vi "day 14 task 1.vi"() -> ()   [LabVIEW 2019]
uses:
  48c75094-737f-452e-9833-d8298e23b8a0.vi
panel:
  out "no. units sand come to rest loop":u32
  out "no. units sand come to rest":u32
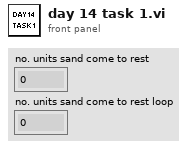
[diagram p1: front panel]
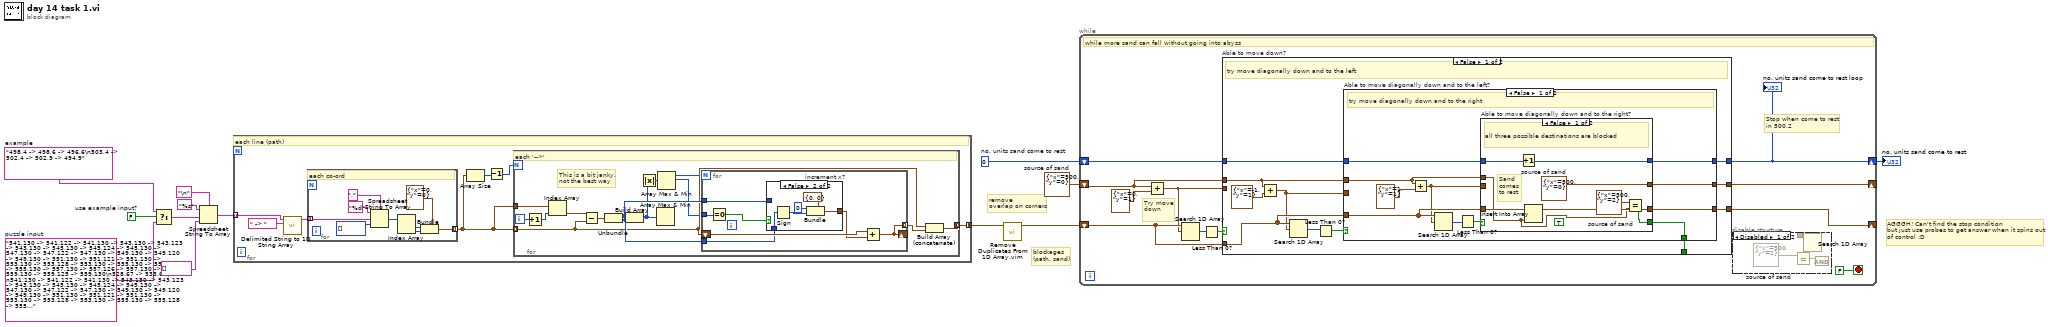
[diagram p0: block diagram]
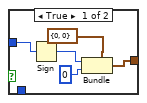
[diagram p6: hidden frame]
diagram:
  w2 = cluster{"x":i32, "y":i32} {"x"=500, "y"=0}  # source of sand
  w3 = u32 0  # no. units sand come to rest
  w8 = FALSE  # use example input?
  w9 = "541,130 -> 541,122 -> 541,130 -> 543,130 -> 543,123 -> 543,130 -> 545,130 -> 545,124 -> 545,130 -> 547,130 -> 547,122 -> 547,130 -> 549,130 -> 549,120 -> 549,130 -> 551,130 -> 551,121 -> 551,130 -> 553,130 -> 553,128 -> 553,130 -> 555,130 -> 555,128 -> 555,130 -> 557,130 -> 557,126 -> 557,130 -> 559,130 -> 559,125 -> 559,130\n528,67 -> 533,67\n541,130 -> 541,122 -> 541,130 -> 543,130 -> 543,123 -> 543,130 -> 545,130 -> 545,124 -> 545,130 -> 547,130 -> 547,122 -> 547,130 -> 549,130 -> 549,120 -> 549,130 -> 551,130 -> 551,121 -> 551,130 -> 553,130 -> 553,128 -> 553,130 -> 555,130 -> 555,128 -> 555,130 -> 557,130 -> 557,126 -> 557,130 -> 559,130 -> 559,125 -> 559,130\n496,23 -> 496,16 -> 496,23 -> 498,23 -> 498,16 -> 498,23 -> 500,23 -> 500,17 -> 500,23 -> 502,23 -> 502,16 -> 502,23\n541,130 -> 541,122 -> 541,130 -> 543,130 -> 543,123 -> 543,130 -> 545,130 -> 545,124 -> 545,130 -> 547,130 -> 547,122 -> 547,130 -> 549,130 -> 549,120 -> 549,130 -> 551,130 -> 551,121 -> 551,130 -> 553,130 -> 553,128 -> 553,130 -> 555,130 -> 555,128 -> 555,130 -> 557,130 -> 557,126 -> 557,130 -> 559,130 -> 559,125 -> 559,130\n514,62 -> 519,62\n509,56 -> 514,56\n497,36 -> 497,30 -> 497,36 -> 499,36 -> 499,27 -> 499,36 -> 501,36 -> 501,33 -> 501,36 -> 503,36 -> 503,27 -> 503,36 -> 505,36 -> 505,28 -> 505,36 -> 507,36 -> 507,35 -> 507,36\n541,130 -> 541,122 -> 541,130 -> 543,130 -> 543,123 -> 543,130 -> 545,130 -> 545,124 -> 545,130 -> 547,130 -> 547,122 -> 547,130 -> 549,130 -> 549,120 -> 549,130 -> 551,130 -> 551,121 -> 551,130 -> 553,130 -> 553,128 -> 553,130 -> 555,130 -> 555,128 -> 555,130 -> 557,130 -> 557,126 -> 557,130 -> 559,130 -> 559,125 -> 559,130\n541,130 -> 541,122 -> 541,130 -> 543,130 -> 543,123 -> 543,130 -> 545,130 -> 545,124 -> 545,130 -> 547,130 -> 547,122 -> 547,130 -> 549,130 -> 549,120 -> 549,130 -> 551,130 -> 551,121 -> 551,130 -> 553,130 -> 553,128 -> 553,130 -> 555,130 -> 555,128 -> 555,130 -> 557,130 -> 557,126 -> 557,130 -> 559,130 -> 559,125 -> 559,130\n574,133 -> 574,137 -> 567,137 -> 567,141 -> 584,141 -> 584,137 -> 576,137 -> 576,133\n524,60 -> 529,60\n574,133 -> 574,137 -> 567,137 -> 567,141 -> 584,141 -> 584,137 -> 576,137 -> 576,133\n541,130 -> 541,122 -> 541,130 -> 543,130 -> 543,123 -> 543,130 -> 545,130 -> 545,124 -> 545,130 -> 547,130 -> 547,122 -> 547,130 -> 549,130 -> 549,120 -> 549,130 -> 551,130 -> 551,121 -> 551,130 -> 553,130 -> 553,128 -> 553,130 -> 555,130 -> 555,128 -> 555,130 -> 557,130 -> 557,126 -> 557,130 -> 559,130 -> 559,125 -> 559,130\n541,130 -> 541,122 -> 541,130 -> 543,130 -> 543,123 -> 543,130 -> 545,130 -> 545,124 -> 545,130 -> 547,130 -> 547,122 -> 547,130 -> 549,130 -> 549,120 -> 549,130 -> 551,130 -> 551,121 -> 551,130 -> 553,130 -> 553,128 -> 553,130 -> 555,130 -> 555,128 -> 555,130 -> 557,130 -> 557,126 -> 557,130 -> 559,130 -> 559,125 -> 559,130\n506,39 -> 506,43 -> 499,43 -> 499,51 -> 514,51 -> 514,43 -> 510,43 -> 510,39\n541,130 -> 541,122 -> 541,130 -> 543,130 -> 543,123 -> 543,130 -> 545,130 -> 545,124 -> 545,130 -> 547,130 -> 547,122 -> 547,130 -> 549,130 -> 549,120 -> 549,130 -> 551,130 -> 551,121 -> 551,130 -> 553,130 -> 553,128 -> 553,130 -> 555,130 -> 555,128 -> 555,130 -> 557,130 -> 557,126 -> 557,130 -> 559,130 -> 559,125 -> 559,130\n541,130 -> 541,122 -> 541,130 -> 543,130 -> 543,123 -> 543,130 -> 545,130 -> 545,124 -> 545,130 -> 547,130 -> 547,122 -> 547,130 -> 549,130 -> 549,120 -> 549,130 -> 551,130 -> 551,121 -> 551,130 -> 553,130 -> 553,128 -> 553,130 -> 555,130 -> 555,128 -> 555,130 -> 557,130 -> 557,126 -> 557,130 -> 559,130 -> 559,125 -> 559,130\n503,60 -> 508,60\n567,115 -> 571,115\n556,151 -> 556,153 -> 548,153 -> 548,157 -> 561,157 -> 561,153 -> 560,153 -> 560,151\n497,36 -> 497,30 -> 497,36 -> 499,36 -> 499,27 -> 499,36 -> 501,36 -> 501,33 -> 501,36 -> 503,36 -> 503,27 -> 503,36 -> 505,36 -> 505,28 -> 505,36 -> 507,36 -> 507,35 -> 507,36\n525,69 -> 530,69\n557,83 -> 557,85 -> 550,85 -> 550,89 -> 569,89 -> 569,85 -> 561,85 -> 561,83\n574,133 -> 574,137 -> 567,137 -> 567,141 -> 584,141 -> 584,137 -> 576,137 -> 576,133\n541,130 -> 541,122 -> 541,130 -> 543,130 -> 543,123 -> 543,130 -> 545,130 -> 545,124 -> 545,130 -> 547,130 -> 547,122 -> 547,130 -> 549,130 -> 549,120 -> 549,130 -> 551,130 -> 551,121 -> 551,130 -> 553,130 -> 553,128 -> 553,130 -> 555,130 -> 555,128 -> 555,130 -> 557,130 -> 557,126 -> 557,130 -> 559,130 -> 559,125 -> 559,130\n496,23 -> 496,16 -> 496,23 -> 498,23 -> 498,16 -> 498,23 -> 500,23 -> 500,17 -> 500,23 -> 502,23 -> 502,16 -> 502,23\n564,108 -> 564,107 -> 564,108 -> 566,108 -> 566,101 -> 566,108 -> 568,108 -> 568,100 -> 568,108\n496,23 -> 496,16 -> 496,23 -> 498,23 -> 498,16 -> 498,23 -> 500,23 -> 500,17 -> 500,23 -> 502,23 -> 502,16 -> 502,23\n556,151 -> 556,153 -> 548,153 -> 548,157 -> 561,157 -> 561,153 -> 560,153 -> 560,151\n541,130 -> 541,122 -> 541,130 -> 543,130 -> 543,123 -> 543,130 -> 545,130 -> 545,124 -> 545,130 -> 547,130 -> 547,122 -> 547,130 -> 549,130 -> 549,120 -> 549,130 -> 551,130 -> 551,121 -> 551,130 -> 553,130 -> 553,128 -> 553,130 -> 555,130 -> 555,128 -> 555,130 -> 557,130 -> 557,126 -> 557,130 -> 559,130 -> 559,125 -> 559,130\n497,36 -> 497,30 -> 497,36 -> 499,36 -> 499,27 -> 499,36 -> 501,36 -> 501,33 -> 501,36 -> 503,36 -> 503,27 -> 503,36 -> 505,36 -> 505,28 -> 505,36 -> 507,36 -> 507,35 -> 507,36\n556,151 -> 556,153 -> 548,153 -> 548,157 -> 561,157 -> 561,153 -> 560,153 -> 560,151\n561,115 -> 565,115\n564,144 -> 568,144\n497,36 -> 497,30 -> 497,36 -> 499,36 -> 499,27 -> 499,36 -> 501,36 -> 501,33 -> 501,36 -> 503,36 -> 503,27 -> 503,36 -> 505,36 -> 505,28 -> 505,36 -> 507,36 -> 507,35 -> 507,36\n541,130 -> 541,122 -> 541,130 -> 543,130 -> 543,123 -> 543,130 -> 545,130 -> 545,124 -> 545,130 -> 547,130 -> 547,122 -> 547,130 -> 549,130 -> 549,120 -> 549,130 -> 551,130 -> 551,121 -> 551,130 -> 553,130 -> 553,128 -> 553,130 -> 555,130 -> 555,128 -> 555,130 -> 557,130 -> 557,126 -> 557,130 -> 559,130 -> 559,125 -> 559,130\n497,36 -> 497,30 -> 497,36 -> 499,36 -> 499,27 -> 499,36 -> 501,36 -> 501,33 -> 501,36 -> 503,36 -> 503,27 -> 503,36 -> 505,36 -> 505,28 -> 505,36 -> 507,36 -> 507,35 -> 507,36\n556,151 -> 556,153 -> 548,153 -> 548,157 -> 561,157 -> 561,153 -> 560,153 -> 560,151\n557,83 -> 557,85 -> 550,85 -> 550,89 -> 569,89 -> 569,85 -> 561,85 -> 561,83\n496,23 -> 496,16 -> 496,23 -> 498,23 -> 498,16 -> 498,23 -> 500,23 -> 500,17 -> 500,23 -> 502,23 -> 502,16 -> 502,23\n567,146 -> 571,146\n531,65 -> 536,65\n528,62 -> 533,62\n541,130 -> 541,122 -> 541,130 -> 543,130 -> 543,123 -> 543,130 -> 545,130 -> 545,124 -> 545,130 -> 547,130 -> 547,122 -> 547,130 -> 549,130 -> 549,120 -> 549,130 -> 551,130 -> 551,121 -> 551,130 -> 553,130 -> 553,128 -> 553,130 -> 555,130 -> 555,128 -> 555,130 -> 557,130 -> 557,126 -> 557,130 -> 559,130 -> 559,125 -> 559,130\n541,130 -> 541,122 -> 541,130 -> 543,130 -> 543,123 -> 543,130 -> 545,130 -> 545,124 -> 545,130 -> 547,130 -> 547,122 -> 547,130 -> 549,130 -> 549,120 -> 549,130 -> 551,130 -> 551,121 -> 551,130 -> 553,130 -> 553,128 -> 553,130 -> 555,130 -> 555,128 -> 555,130 -> 557,130 -> 557,126 -> 557,130 -> 559,130 -> 559,125 -> 559,130\n574,133 -> 574,137 -> 567,137 -> 567,141 -> 584,141 -> 584,137 -> 576,137 -> 576,133\n568,95 -> 571,95 -> 571,94\n497,36 -> 497,30 -> 497,36 -> 499,36 -> 499,27 -> 499,36 -> 501,36 -> 501,33 -> 501,36 -> 503,36 -> 503,27 -> 503,36 -> 505,36 -> 505,28 -> 505,36 -> 507,36 -> 507,35 -> 507,36\n497,36 -> 497,30 -> 497,36 -> 499,36 -> 499,27 -> 499,36 -> 501,36 -> 501,33 -> 501,36 -> 503,36 -> 503,27 -> 503,36 -> 505,36 -> 505,28 -> 505,36 -> 507,36 -> 507,35 -> 507,36\n497,36 -> 497,30 -> 497,36 -> 499,36 -> 499,27 -> 499,36 -> 501,36 -> 501,33 -> 501,36 -> 503,36 -> 503,27 -> 503,36 -> 505,36 -> 505,28 -> 505,36 -> 507,36 -> 507,35 -> 507,36\n541,130 -> 541,122 -> 541,130 -> 543,130 -> 543,123 -> 543,130 -> 545,130 -> 545,124 -> 545,130 -> 547,130 -> 547,122 -> 547,130 -> 549,130 -> 549,120 -> 549,130 -> 551,130 -> 551,121 -> 551,130 -> 553,130 -> 553,128 -> 553,130 -> 555,130 -> 555,128 -> 555,130 -> 557,130 -> 557,126 -> 557,130 -> 559,130 -> 559,125 -> 559,130\n557,83 -> 557,85 -> 550,85 -> 550,89 -> 569,89 -> 569,85 -> 561,85 -> 561,83\n543,72 -> 543,73 -> 554,73 -> 554,72\n506,39 -> 506,43 -> 499,43 -> 499,51 -> 514,51 -> 514,43 -> 510,43 -> 510,39\n555,115 -> 559,115\n496,23 -> 496,16 -> 496,23 -> 498,23 -> 498,16 -> 498,23 -> 500,23 -> 500,17 -> 500,23 -> 502,23 -> 502,16 -> 502,23\n506,39 -> 506,43 -> 499,43 -> 499,51 -> 514,51 -> 514,43 -> 510,43 -> 510,39\n536,75 -> 536,76 -> 547,76 -> 547,75\n521,62 -> 526,62\n564,108 -> 564,107 -> 564,108 -> 566,108 -> 566,101 -> 566,108 -> 568,108 -> 568,100 -> 568,108\n574,133 -> 574,137 -> 567,137 -> 567,141 -> 584,141 -> 584,137 -> 576,137 -> 576,133\n516,56 -> 521,56\n564,108 -> 564,107 -> 564,108 -> 566,108 -> 566,101 -> 566,108 -> 568,108 -> 568,100 -> 568,108\n543,72 -> 543,73 -> 554,73 -> 554,72\n574,133 -> 574,137 -> 567,137 -> 567,141 -> 584,141 -> 584,137 -> 576,137 -> 576,133\n564,113 -> 568,113\n506,39 -> 506,43 -> 499,43 -> 499,51 -> 514,51 -> 514,43 -> 510,43 -> 510,39\n541,130 -> 541,122 -> 541,130 -> 543,130 -> 543,123 -> 543,130 -> 545,130 -> 545,124 -> 545,130 -> 547,130 -> 547,122 -> 547,130 -> 549,130 -> 549,120 -> 549,130 -> 551,130 -> 551,121 -> 551,130 -> 553,130 -> 553,128 -> 553,130 -> 555,130 -> 555,128 -> 555,130 -> 557,130 -> 557,126 -> 557,130 -> 559,130 -> 559,125 -> 559,130\n496,23 -> 496,16 -> 496,23 -> 498,23 -> 498,16 -> 498,23 -> 500,23 -> 500,17 -> 500,23 -> 502,23 -> 502,16 -> 502,23\n557,83 -> 557,85 -> 550,85 -> 550,89 -> 569,89 -> 569,85 -> 561,85 -> 561,83\n558,113 -> 562,113\n497,36 -> 497,30 -> 497,36 -> 499,36 -> 499,27 -> 499,36 -> 501,36 -> 501,33 -> 501,36 -> 503,36 -> 503,27 -> 503,36 -> 505,36 -> 505,28 -> 505,36 -> 507,36 -> 507,35 -> 507,36\n506,39 -> 506,43 -> 499,43 -> 499,51 -> 514,51 -> 514,43 -> 510,43 -> 510,39\n497,36 -> 497,30 -> 497,36 -> 499,36 -> 499,27 -> 499,36 -> 501,36 -> 501,33 -> 501,36 -> 503,36 -> 503,27 -> 503,36 -> 505,36 -> 505,28 -> 505,36 -> 507,36 -> 507,35 -> 507,36\n568,95 -> 571,95 -> 571,94\n497,36 -> 497,30 -> 497,36 -> 499,36 -> 499,27 -> 499,36 -> 501,36 -> 501,33 -> 501,36 -> 503,36 -> 503,27 -> 503,36 -> 505,36 -> 505,28 -> 505,36 -> 507,36 -> 507,35 -> 507,36\n510,60 -> 515,60\n497,36 -> 497,30 -> 497,36 -> 499,36 -> 499,27 -> 499,36 -> 501,36 -> 501,33 -> 501,36 -> 503,36 -> 503,27 -> 503,36 -> 505,36 -> 505,28 -> 505,36 -> 507,36 -> 507,35 -> 507,36\n557,83 -> 557,85 -> 550,85 -> 550,89 -> 569,89 -> 569,85 -> 561,85 -> 561,83\n570,117 -> 574,117\n497,36 -> 497,30 -> 497,36 -> 499,36 -> 499,27 -> 499,36 -> 501,36 -> 501,33 -> 501,36 -> 503,36 -> 503,27 -> 503,36 -> 505,36 -> 505,28 -> 505,36 -> 507,36 -> 507,35 -> 507,36\n507,62 -> 512,62\n541,130 -> 541,122 -> 541,130 -> 543,130 -> 543,123 -> 543,130 -> 545,130 -> 545,124 -> 545,130 -> 547,130 -> 547,122 -> 547,130 -> 549,130 -> 549,120 -> 549,130 -> 551,130 -> 551,121 -> 551,130 -> 553,130 -> 553,128 -> 553,130 -> 555,130 -> 555,128 -> 555,130 -> 557,130 -> 557,126 -> 557,130 -> 559,130 -> 559,125 -> 559,130\n556,151 -> 556,153 -> 548,153 -> 548,157 -> 561,157 -> 561,153 -> 560,153 -> 560,151\n564,108 -> 564,107 -> 564,108 -> 566,108 -> 566,101 -> 566,108 -> 568,108 -> 568,100 -> 568,108\n541,130 -> 541,122 -> 541,130 -> 543,130 -> 543,123 -> 543,130 -> 545,130 -> 545,124 -> 545,130 -> 547,130 -> 547,122 -> 547,130 -> 549,130 -> 549,120 -> 549,130 -> 551,130 -> 551,121 -> 551,130 -> 553,130 -> 553,128 -> 553,130 -> 555,130 -> 555,128 -> 555,130 -> 557,130 -> 557,126 -> 557,130 -> 559,130 -> 559,125 -> 559,130\n506,39 -> 506,43 -> 499,43 -> 499,51 -> 514,51 -> 514,43 -> 510,43 -> 510,39\n564,108 -> 564,107 -> 564,108 -> 566,108 -> 566,101 -> 566,108 -> 568,108 -> 568,100 -> 568,108\n497,36 -> 497,30 -> 497,36 -> 499,36 -> 499,27 -> 499,36 -> 501,36 -> 501,33 -> 501,36 -> 503,36 -> 503,27 -> 503,36 -> 505,36 -> 505,28 -> 505,36 -> 507,36 -> 507,35 -> 507,36\n561,111 -> 565,111\n541,130 -> 541,122 -> 541,130 -> 543,130 -> 543,123 -> 543,130 -> 545,130 -> 545,124 -> 545,130 -> 547,130 -> 547,122 -> 547,130 -> 549,130 -> 549,120 -> 549,130 -> 551,130 -> 551,121 -> 551,130 -> 553,130 -> 553,128 -> 553,130 -> 555,130 -> 555,128 -> 555,130 -> 557,130 -> 557,126 -> 557,130 -> 559,130 -> 559,125 -> 559,130\n541,130 -> 541,122 -> 541,130 -> 543,130 -> 543,123 -> 543,130 -> 545,130 -> 545,124 -> 545,130 -> 547,130 -> 547,122 -> 547,130 -> 549,130 -> 549,120 -> 549,130 -> 551,130 -> 551,121 -> 551,130 -> 553,130 -> 553,128 -> 553,130 -> 555,130 -> 555,128 -> 555,130 -> 557,130 -> 557,126 -> 557,130 -> 559,130 -> 559,125 -> 559,130\n541,130 -> 541,122 -> 541,130 -> 543,130 -> 543,123 -> 543,130 -> 545,130 -> 545,124 -> 545,130 -> 547,130 -> 547,122 -> 547,130 -> 549,130 -> 549,120 -> 549,130 -> 551,130 -> 551,121 -> 551,130 -> 553,130 -> 553,128 -> 553,130 -> 555,130 -> 555,128 -> 555,130 -> 557,130 -> 557,126 -> 557,130 -> 559,130 -> 559,125 -> 559,130\n496,23 -> 496,16 -> 496,23 -> 498,23 -> 498,16 -> 498,23 -> 500,23 -> 500,17 -> 500,23 -> 502,23 -> 502,16 -> 502,23\n558,148 -> 562,148\n513,58 -> 518,58\n564,108 -> 564,107 -> 564,108 -> 566,108 -> 566,101 -> 566,108 -> 568,108 -> 568,100 -> 568,108\n558,117 -> 562,117\n557,83 -> 557,85 -> 550,85 -> 550,89 -> 569,89 -> 569,85 -> 561,85 -> 561,83\n546,79 -> 546,80 -> 558,80\n541,130 -> 541,122 -> 541,130 -> 543,130 -> 543,123 -> 543,130 -> 545,130 -> 545,124 -> 545,130 -> 547,130 -> 547,122 -> 547,130 -> 549,130 -> 549,120 -> 549,130 -> 551,130 -> 551,121 -> 551,130 -> 553,130 -> 553,128 -> 553,130 -> 555,130 -> 555,128 -> 555,130 -> 557,130 -> 557,126 -> 557,130 -> 559,130 -> 559,125 -> 559,130\n541,130 -> 541,122 -> 541,130 -> 543,130 -> 543,123 -> 543,130 -> 545,130 -> 545,124 -> 545,130 -> 547,130 -> 547,122 -> 547,130 -> 549,130 -> 549,120 -> 549,130 -> 551,130 -> 551,121 -> 551,130 -> 553,130 -> 553,128 -> 553,130 -> 555,130 -> 555,128 -> 555,130 -> 557,130 -> 557,126 -> 557,130 -> 559,130 -> 559,125 -> 559,130\n536,75 -> 536,76 -> 547,76 -> 547,75\n500,62 -> 505,62\n506,39 -> 506,43 -> 499,43 -> 499,51 -> 514,51 -> 514,43 -> 510,43 -> 510,39\n556,151 -> 556,153 -> 548,153 -> 548,157 -> 561,157 -> 561,153 -> 560,153 -> 560,151\n520,58 -> 525,58\n535,67 -> 540,67\n574,133 -> 574,137 -> 567,137 -> 567,141 -> 584,141 -> 584,137 -> 576,137 -> 576,133\n497,36 -> 497,30 -> 497,36 -> 499,36 -> 499,27 -> 499,36 -> 501,36 -> 501,33 -> 501,36 -> 503,36 -> 503,27 -> 503,36 -> 505,36 -> 505,28 -> 505,36 -> 507,36 -> 507,35 -> 507,36\n541,130 -> 541,122 -> 541,130 -> 543,130 -> 543,123 -> 543,130 -> 545,130 -> 545,124 -> 545,130 -> 547,130 -> 547,122 -> 547,130 -> 549,130 -> 549,120 -> 549,130 -> 551,130 -> 551,121 -> 551,130 -> 553,130 -> 553,128 -> 553,130 -> 555,130 -> 555,128 -> 555,130 -> 557,130 -> 557,126 -> 557,130 -> 559,130 -> 559,125 -> 559,130\n546,79 -> 546,80 -> 558,80\n564,108 -> 564,107 -> 564,108 -> 566,108 -> 566,101 -> 566,108 -> 568,108 -> 568,100 -> 568,108\n543,72 -> 543,73 -> 554,73 -> 554,72\n564,117 -> 568,117\n497,36 -> 497,30 -> 497,36 -> 499,36 -> 499,27 -> 499,36 -> 501,36 -> 501,33 -> 501,36 -> 503,36 -> 503,27 -> 503,36 -> 505,36 -> 505,28 -> 505,36 -> 507,36 -> 507,35 -> 507,36\n497,36 -> 497,30 -> 497,36 -> 499,36 -> 499,27 -> 499,36 -> 501,36 -> 501,33 -> 501,36 -> 503,36 -> 503,27 -> 503,36 -> 505,36 -> 505,28 -> 505,36 -> 507,36 -> 507,35 -> 507,36\n536,75 -> 536,76 -> 547,76 -> 547,75\n557,83 -> 557,85 -> 550,85 -> 550,89 -> 569,89 -> 569,85 -> 561,85 -> 561,83\n496,23 -> 496,16 -> 496,23 -> 498,23 -> 498,16 -> 498,23 -> 500,23 -> 500,17 -> 500,23 -> 502,23 -> 502,16 -> 502,23\n541,130 -> 541,122 -> 541,130 -> 543,130 -> 543,123 -> 543,130 -> 545,130 -> 545,124 -> 545,130 -> 547,130 -> 547,122 -> 547,130 -> 549,130 -> 549,120 -> 549,130 -> 551,130 -> 551,121 -> 551,130 -> 553,130 -> 553,128 -> 553,130 -> 555,130 -> 555,128 -> 555,130 -> 557,130 -> 557,126 -> 557,130 -> 559,130 -> 559,125 -> 559,130\n539,69 -> 544,69\n552,117 -> 556,117\n556,151 -> 556,153 -> 548,153 -> 548,157 -> 561,157 -> 561,153 -> 560,153 -> 560,151\n496,23 -> 496,16 -> 496,23 -> 498,23 -> 498,16 -> 498,23 -> 500,23 -> 500,17 -> 500,23 -> 502,23 -> 502,16 -> 502,23\n561,146 -> 565,146\n570,148 -> 574,148\n496,23 -> 496,16 -> 496,23 -> 498,23 -> 498,16 -> 498,23 -> 500,23 -> 500,17 -> 500,23 -> 502,23 -> 502,16 -> 502,23\n496,23 -> 496,16 -> 496,23 -> 498,23 -> 498,16 -> 498,23 -> 500,23 -> 500,17 -> 500,23 -> 502,23 -> 502,16 -> 502,23\n532,69 -> 537,69\n564,108 -> 564,107 -> 564,108 -> 566,108 -> 566,101 -> 566,108 -> 568,108 -> 568,100 -> 568,108\n512,54 -> 517,54\n541,130 -> 541,122 -> 541,130 -> 543,130 -> 543,123 -> 543,130 -> 545,130 -> 545,124 -> 545,130 -> 547,130 -> 547,122 -> 547,130 -> 549,130 -> 549,120 -> 549,130 -> 551,130 -> 551,121 -> 551,130 -> 553,130 -> 553,128 -> 553,130 -> 555,130 -> 555,128 -> 555,130 -> 557,130 -> 557,126 -> 557,130 -> 559,130 -> 559,125 -> 559,130\n541,130 -> 541,122 -> 541,130 -> 543,130 -> 543,123 -> 543,130 -> 545,130 -> 545,124 -> 545,130 -> 547,130 -> 547,122 -> 547,130 -> 549,130 -> 549,120 -> 549,130 -> 551,130 -> 551,121 -> 551,130 -> 553,130 -> 553,128 -> 553,130 -> 555,130 -> 555,128 -> 555,130 -> 557,130 -> 557,126 -> 557,130 -> 559,130 -> 559,125 -> 559,130\n517,60 -> 522,60\n564,148 -> 568,148\n506,58 -> 511,58\n541,130 -> 541,122 -> 541,130 -> 543,130 -> 543,123 -> 543,130 -> 545,130 -> 545,124 -> 545,130 -> 547,130 -> 547,122 -> 547,130 -> 549,130 -> 549,120 -> 549,130 -> 551,130 -> 551,121 -> 551,130 -> 553,130 -> 553,128 -> 553,130 -> 555,130 -> 555,128 -> 555,130 -> 557,130 -> 557,126 -> 557,130 -> 559,130 -> 559,125 -> 559,130\n541,130 -> 541,122 -> 541,130 -> 543,130 -> 543,123 -> 543,130 -> 545,130 -> 545,124 -> 545,130 -> 547,130 -> 547,122 -> 547,130 -> 549,130 -> 549,120 -> 549,130 -> 551,130 -> 551,121 -> 551,130 -> 553,130 -> 553,128 -> 553,130 -> 555,130 -> 555,128 -> 555,130 -> 557,130 -> 557,126 -> 557,130 -> 559,130 -> 559,125 -> 559,130"  # puzzle input
  w10 = "498,4 -> 498,6 -> 496,6\n503,4 -> 502,4 -> 502,9 -> 494,9"  # example
  # "AGGGH! Can't find the stop condition \nbut just use probes to get answer when it spins out\nof control :D"
  # "blockages\n(path, sand)"
  # "remove\noverlap on corners"
  n1 = Select(t=w10, s=w8, f=w9) -> (s? t:f=w7:string)
  n2 = Spreadsheet String To Array(delimiter (Tab)="\n", format string="%s", spreadsheet string=w7, array type (2D Dbl)=string[] []) -> (array=w6:string[])
  n3 = for {
    tunnel: w6 -> [w20] mode=indexing
    tunnel: [w14] -> w5 mode=concatenating
    # "each line (path)"
    n4 = call <vilib>:"Delimited String to 1D String Array.vi"("delimiter"=" -> ", "delimited string"=w20) -> ("string array"=w18:string[])  [unwired: 9 in]
    n5 = for {
      tunnel: w18 -> [w57] mode=indexing
      tunnel: [w52] -> w15 mode=indexing
      # "each co-ord"
      n6 = Spreadsheet String To Array(delimiter (Tab)=",", format string="%d", spreadsheet string=w57, array type (2D Dbl)=i32[] []) -> (array=w56:i32[])
      n7 = Index Array(array=w56) -> (element #1=w55:i32, element #2=w54:i32)  [unwired: 2 in]
      n8 = Bundle(cluster=cluster{"x":i32, "y":i32} {"x"=0, "y"=0}, "x"=w55, "y"=w54) -> (w52:cluster{"x":i32, "y":i32})
    }
    n9 = Array Size(array=w15) -> (size(s)=w16:i32)
    n10 = Decrement(x=w16) -> (x-1=w17:i32)
    n11 = for {
      N: w17 -> [_]
      tunnel: w15 -> [w26] mode=indexing
      tunnel: w15 -> [w34]
      tunnel: [w27] -> w14 mode=concatenating
      i -> [w33]
      # "This is a bit janky, \nnot the best way"
      # "each '-->'"
      n12 = Increment(x=w33) -> (x+1=w32:i32)
      n13 = Index Array(array=w34, index=w32) -> (element=w28:cluster{"x":i32, "y":i32})
      n14 = Subtract(x=w28, y=w26) -> (x-y=w31:cluster{"x":i32, "y":i32})
      n15 = Unbundle(w31) -> ("x"=w30:i32, "y"=w29:i32)
      n16 = Build Array(w30, w29) -> (w24:i32[])
      n17 = Absolute Value(x=w24) -> (abs(x)=w23:i32[])
      n18 = Array Max & Min(array=w24) -> ()  [unwired: 4 out]
      n19 = Array Max & Min(array=w23) -> (max value=w22:i32, max index (indices)=w21:i32)  [unwired: 2 out]
      n20 = for {
        N: w22 -> [_]
        tunnel: w21 -> [w41]
        tunnel: w30 -> [w36]
        shift-right: [w37] -> _
        shift-left: w26 -> [w40]
        tunnel: [w37] -> w25 mode=indexing
        tunnel: w29 -> [w35]
        n21 = Equal To 0?(x=w41) -> (x = 0?=w38:bool)
        n22 = case "increment x?" shown="False" w38 {
          tunnel: [w44 w50] -> w39
          tunnel: w36 -> [w43 _]
          tunnel: w35 -> [_ w47]
          frame True {
            n23 = Sign(1:w43) -> (0:w42:i32)
            n24 = Bundle(cluster=cluster{"x":i32, "y":i32} {"x"=0, "y"=0}, "x"=w42, "y"=0) -> (w44:cluster{"x":i32, "y":i32})
          }
          frame False {
            n25 = Sign(1:w47) -> (0:w48:i32)
            n26 = Bundle(cluster=cluster{"x":i32, "y":i32} {"x"=0, "y"=0}, "x"=0 ("y"), "y"=w48) -> (w50:cluster{"x":i32, "y":i32})
          }
        }
        n27 = Add(x=w40, y=w39) -> (x+y=w37:cluster{"x":i32, "y":i32})
      }
      n28 = Build Array (concatenate)(w26, w25) -> (w27:cluster{"x":i32, "y":i32}[])
    }
  }
  n29 = call "Remove Duplicates From 1D Array.vim"("array"=w5) -> ("array with duplicates removed"=w4:cluster{"x":i32, "y":i32}[])  [unwired: 10 in]
  n30 = while {
    shift-right: [w63] -> _
    shift-left: w2 -> [w67]
    shift-right: [w65] -> w1
    shift-left: w3 -> [w68]
    shift-right: [w62] -> _
    shift-left: w4 -> [w66]
    stop <- FALSE stop-if-true
    # "Stop when come to rest\nin 500,2"
    # "Try move down"
    # "while more sand can fall without going into abyss"
    n31 = Add(x=w67, y=cluster{"x":i32, "y":i32} {"x"=0, "y"=1} ("source of sand")) -> (x+y=w64:cluster{"x":i32, "y":i32})
    n32 = Search 1D Array(1D array=w66, element=w64) -> (index of element=w70:i32)  [unwired: 1 in]
    n33 = Less Than 0?(x=w70) -> (x < 0?=w69:bool)
    n34 = case "Able to move down?" shown="False" w69 {
      tunnel: w68 -> [w80 w113]
      tunnel: w67 -> [w81 _]
      tunnel: w66 -> [w82 w111]
      tunnel: [w79 w113] -> w65
      tunnel: [w77 w112] -> w63
      tunnel: [w76 w111] -> w62
      tunnel: w64 -> [_ w112]
      tunnel: [w75 _] -> _
      frame False {
        # "try move diagonally down and to the left"
        n35 = Add(x=w81, y=cluster{"x":i32, "y":i32} {"x"=-1, "y"=1} ("source of sand")) -> (x+y=w78:cluster{"x":i32, "y":i32})
        n36 = Search 1D Array(1D array=w82, element=w78) -> (index of element=w84:i32)  [unwired: 1 in]
        n37 = Less Than 0?(x=w84) -> (x < 0?=w83:bool)
        n38 = case "Able to move diagonally down and to the left?" shown="False" w83 {
          tunnel: w82 -> [w91 w108]
          tunnel: w81 -> [w90 _]
          tunnel: w80 -> [w93 w110]
          tunnel: [w92 w110] -> w79
          tunnel: w78 -> [_ w109]
          tunnel: [w88 w109] -> w77
          tunnel: [w89 w108] -> w76
          tunnel: [w86 _] -> w75
          frame False {
            # "try move diagonally down and to the right"
            n39 = Add(x=w90, y=cluster{"x":i32, "y":i32} {"x"=1, "y"=1} ("source of sand")) -> (x+y=w87:cluster{"x":i32, "y":i32})
            n40 = Search 1D Array(1D array=w91, element=w87) -> (index of element=w95:i32)  [unwired: 1 in]
            n41 = Less Than 0?(x=w95) -> (x < 0?=w94:bool)
            n42 = case "Able to move diagonally down and to the right?" shown="False" w94 {
              tunnel: w93 -> [w104 w105]
              tunnel: [w103 w105] -> w92
              tunnel: w91 -> [w102 w106]
              tunnel: w90 -> [w97 _]
              tunnel: [w101 w106] -> w89
              tunnel: [w100 w107] -> w88
              tunnel: w87 -> [_ w107]
              tunnel: [w99 _] -> w86
              frame False {
                w98 = cluster{"x":i32, "y":i32} {"x"=500, "y"=2}  # source of sand
                (unwired) TRUE
                w100 = cluster{"x":i32, "y":i32} {"x"=500, "y"=0}  # source of sand
                # "Sand comes to rest"
                # "all three possible destinations are blocked"
                n43 = Increment(x=w104) -> (x+1=w103:u32)
                n44 = Insert Into Array(array=w102, new element=w97) -> (w101:cluster{"x":i32, "y":i32}[])  [unwired: 1 in]
                n45 = Equal?(x=w98, y=w97) -> (x = y?=w99:bool)
              }
              frame True {
                # "make move"
              }
            }
          }
          frame True {
            # "use this position for next turn"
          }
        }
      }
      frame True {
        # "use this position for next turn"
      }
    }
    "no. units sand come to rest loop" <- w65
    n46 = disable-structure shown="Disabled" {
      disable-tunnel: _ -> [w72 _]
      frame Disabled {
        w73 = cluster{"x":i32, "y":i32} {"x"=500, "y"=2}  # source of sand
        n47 = Equal?(x=w73) -> (x = y?=w74:bool)  [unwired: 1 in]
        n48 = Search 1D Array(1D array=w72) -> ()  [unwired: 2 in, 1 out]
        n49 = And(x=w74) -> ()  [unwired: 1 in, 1 out]
      }
      frame Enabled {
      }
    }
  }
  "no. units sand come to rest" <- w1
